vi "Flush Data to Log File.vi"(8 "error in (no error)":errorcluster, 10 "Data Queue":refnum<queue>, 11 "Settings in":T1) -> (0 "error out":errorcluster, 3 "Settings out":T1)   [LabVIEW 2021, in "Logging.lvlib"]
doc: "Flush the data queue of any pending data and write it to the data log file."
uses:
  Logging.lvlib
  controls/Acquired Data.ctl
  Settings/Settings.ctl
  Acquisition/Hardware Configuration.ctl
  Acquisition/Channel Settings.ctl
  Acquisition/IO Device.ctl
  Interval Timer/Repeat Interval.ctl
  Interval Timer/Interval Length.ctl
  Interval Timer/Interval Token.ctl
  Logging Configuration.ctl
  Diagnostics/Diagnostics Configuration.ctl
  Acquisition/Acquisition.lvlib
  Settings/Settings.lvlib
  Interval Timer/Interval Timer.lvlib
  Diagnostics/Diagnostics.lvlib
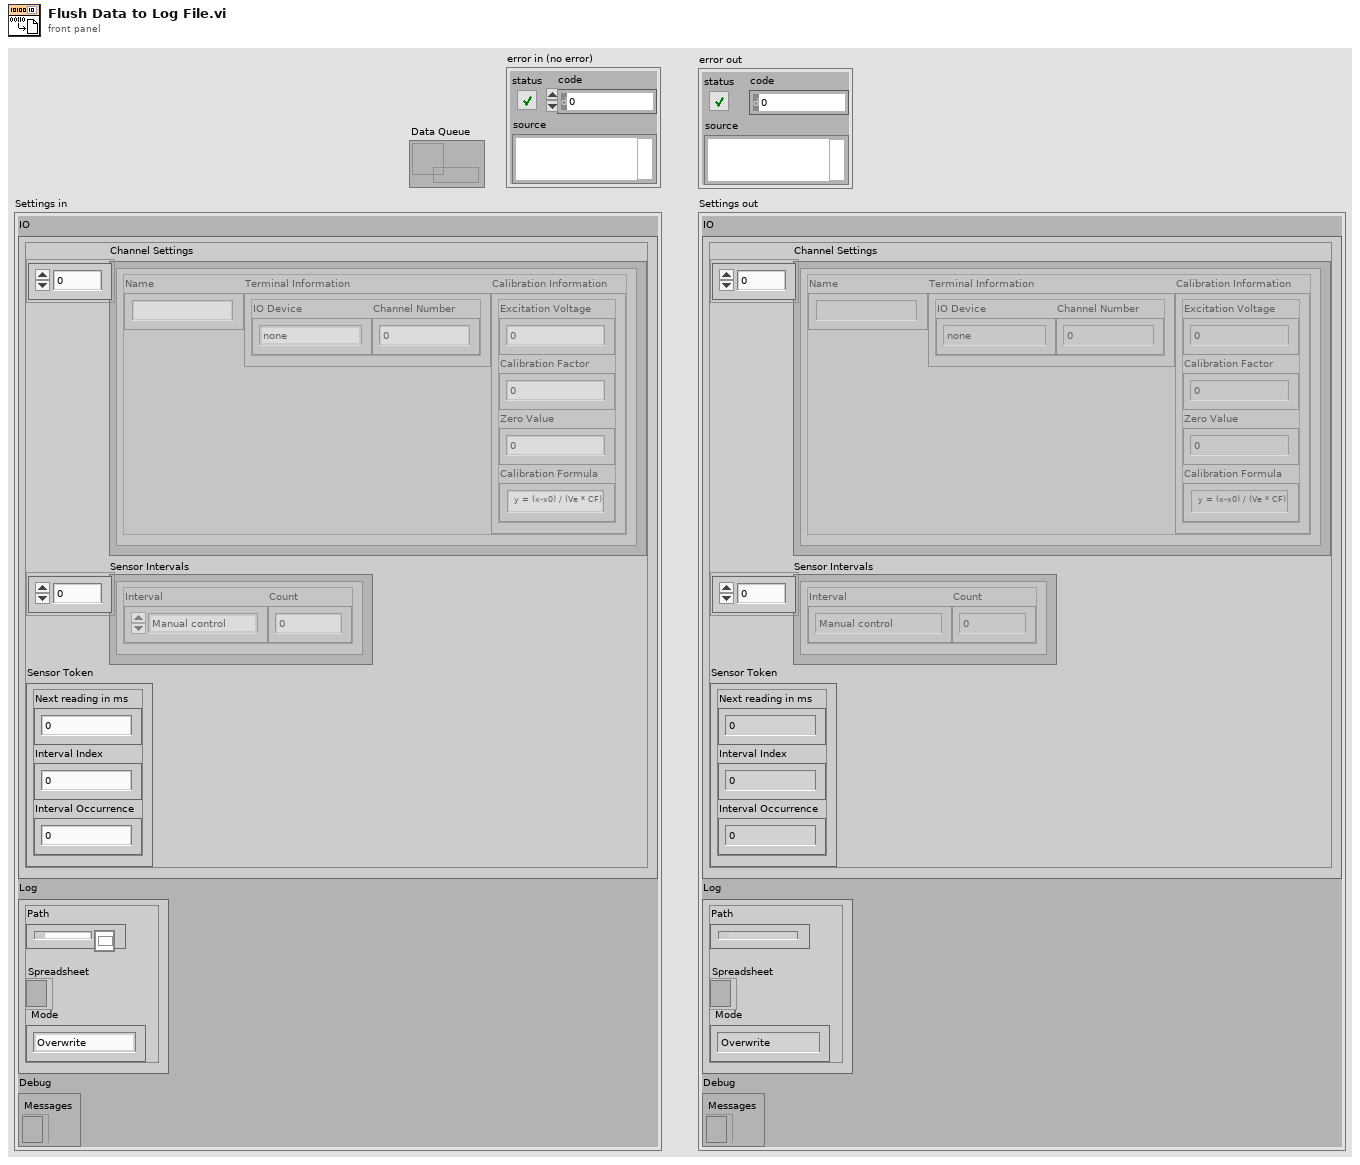
[diagram p1: front panel]
types:
  T1 = typedef "Settings.lvlib/Settings.ctl" = cluster{"IO":T2, "Log":T8, "Debug":T9}
  T2 = typedef "Acquisition.lvlib/Hardware Configuration.ctl" = cluster{"Channel Settings":T3[], "Sensor Intervals":T5[], "Sensor Token":T7}
  T3 = typedef "Acquisition.lvlib/Channel Settings.ctl" = cluster{"Name":string, "Terminal Information":cluster{"IO Device":T4, "Channel Number":i32}, "Calibration Information":cluster{"Excitation Voltage":dbl, "Calibration Factor":dbl, "Zero Value":dbl, "Calibration Formula":string}}
  T4 = typedef "Acquisition.lvlib/IO Device.ctl" = enum16{"none", "9219", "9401"}
  T5 = typedef "Interval Timer.lvlib/Repeat Interval.ctl" = cluster{"Interval":T6, "Count":i32}
  T6 = typedef "Interval Timer.lvlib/Interval Length.ctl" = enum16{"Manual control", "1 second", "10 seconds", "30 seconds", "60 seconds", "600 seconds", "1200 seconds", "3600 seconds"}
  T7 = typedef "Interval Timer.lvlib/Interval Token.ctl" = cluster{"Next reading in ms":u32, "Interval Index":i32, "Interval Occurrence":i32}
  T8 = typedef "Logging.lvlib/Logging Configuration.ctl" = cluster{"Path":path, "Spreadsheet":refnum<file>, "Mode":enum16{"Overwrite", "Append", "Create New"}}
  T9 = typedef "Diagnostics.lvlib/Diagnostics Configuration.ctl" = cluster{"Messages":refnum<file>}
  T10 = typedef "Acquired Data.ctl" = cluster{"Waveform Array":waveform(dbl)[]}
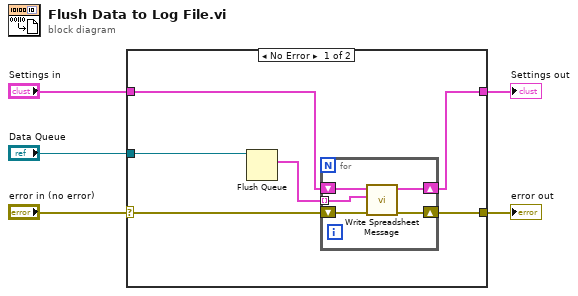
[diagram p0: block diagram]
diagram:
  n1 = case shown="No Error" "error in (no error)" {
    selector: "error in (no error)" -> [w9 w18]
    tunnel: "Data Queue" -> [w10 _]
    tunnel: "Settings in" -> [w8 w17]
    tunnel: [w7 w18] -> w3
    tunnel: [w6 w17] -> w1
    frame No Error {
      n2 = Flush Queue(queue=w10) -> (remaining elements=w11:T10[])  [unwired: 1 in, 2 out]
      n3 = for {
        shift-right: [w15] -> w6
        shift-left: w8 -> [w16]
        shift-right: [w12] -> w7
        shift-left: w9 -> [w13]
        tunnel: w11 -> [w14] mode=indexing
        n4 = call "Write Spreadsheet Message.vi"("error in (no error)"=w13, "Acquired Data"=w14, "Settings"=w16) -> ("error out"=w12:errorcluster, "Settings"=w15:T1)  [unwired: 7 in]
      }
    }
    frame Error {
    }
  }
  "error out" <- w3
  "Settings out" <- w1
